vi "GetFPGAPersonalityDescription.vi"(8 "error in (no error)":errorcluster, 10 "FPGA Personality Name":string, 11 "ProdID":u32) -> (0 "error out":errorcluster, 1 "Help Link":string, 2 "CHM Link":string, 3 "Description":string, 5 "IO Info":T1[](array[typedef]))   [LabVIEW 2021, in "myRIOMetaDataObj.lvclass"]
uses:
  myRIOMetaDataObj.lvclass
  IODetail.ctl
  <vilib>/myRIO/Common/FPGA Personality Framework/Personality.lvlib
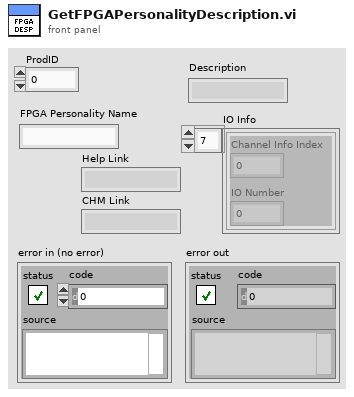
[diagram p1: front panel]
types:
  T1 = typedef "myRIOMetaDataObj.lvclass/IODetail.ctl" = cluster{"Channel Info Index":i8, "IO Number":i8}
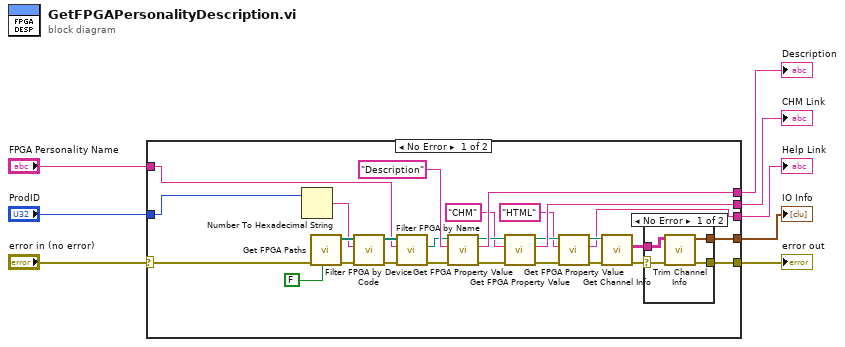
[diagram p0: block diagram]
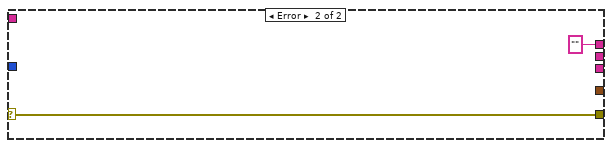
[diagram p3: hidden frame]
diagram:
  n1 = case shown="No Error" "error in (no error)" {
    selector: "error in (no error)" -> [w35 w42]
    tunnel: "ProdID" -> [w9 _]
    tunnel: [w23 w42] -> w5
    tunnel: [w27 "" ("Property Value")] -> w7
    tunnel: "FPGA Personality Name" -> [w26 _]
    tunnel: [w24 _] -> w4
    tunnel: [w18 _] -> w3
    tunnel: [w12 _] -> w2
    frame No Error {
      n2 = Number To Hexadecimal String(2:w9) -> (0:w11:string)  [unwired: 1 in]
      n3 = call <vilib>:"Get FPGA Paths.vi"("Filter Customized (T)"=FALSE, "error in (no error)"=w35) -> ("error out"=w33:errorcluster, "FPGA Personality File Paths"=w34:path[])  [unwired: 8 in]
      n4 = call <vilib>:"Filter FPGA by Device Code.vi"("error in (no error)"=w33, "Device Code"=w11, "FPGA Personality File Paths"=w34) -> ("error out"=w31:errorcluster, "Filtered FPGA Personality File Paths"=w32:path[])  [unwired: 7 in]
      n5 = call <vilib>:"Filter FPGA by Name.vi"("error in (no error)"=w31, "FPGA Personality Name"=w26, "FPGA Personality File Paths"=w32) -> ("error out"=w28:errorcluster, "First Path"=w29:path)  [unwired: 6 in, 1 out]
      n6 = call <vilib>:"Get FPGA Property Value.vi"("error in (no error)"=w28, "Property Name"="Description", "FPGA Personality File Path"=w29) -> ("error out"=w21:errorcluster, "Property Value"=w27:string, "Duplicated FPGA Personality File Path"=w20:path)  [unwired: 5 in, 1 out]
      n7 = call <vilib>:"Get FPGA Property Value.vi"("error in (no error)"=w21, "Property Name"="CHM", "FPGA Personality File Path"=w20) -> ("error out"=w17:errorcluster, "Property Value"=w18:string, "Duplicated FPGA Personality File Path"=w14:path)  [unwired: 5 in, 1 out]
      n8 = call <vilib>:"Get FPGA Property Value.vi"("error in (no error)"=w17, "Property Name"="HTML", "FPGA Personality File Path"=w14) -> ("error out"=w16:errorcluster, "Property Value"=w12:string, "Duplicated FPGA Personality File Path"=w15:path)  [unwired: 5 in, 1 out]
      n9 = call <vilib>:"Get Channel Info.vi"("error in (no error)"=w16, "FPGA Personality File Path"=w15) -> ("error out"=w25:errorcluster, "Channel Info"=w22:string[][])  [unwired: 7 in, 1 out]
      n10 = case shown="No Error" w25 {
        selector: w25 -> [w39 w40]
        tunnel: [w37 _] -> w24
        tunnel: [w38 w40] -> w23
        tunnel: w22 -> [w36 _]
        frame No Error {
          n11 = call "Trim Channel Info.vi"("error IO"=w39, "Raw Channel Info"=w36) -> ("error out"=w38:errorcluster, "Trimmed Channel Info"=w37:T1[])  [unwired: 8 in]
        }
        frame Error {
        }
      }
    }
    frame Error {
    }
  }
  "error out" <- w5
  "Description" <- w7
  "IO Info" <- w4
  "Help Link" <- w2
  "CHM Link" <- w3
